vi "Quick Stack Get and Write Image.vi"(0 "Notifier Name":string, 7 "Write File Ref":refnum<file>, 11 "Num of Frames":u16) -> ()   [LabVIEW 2016]
uses:
  Device Library/Cameras/Camera Controls/Generic Camera Actions.ctl
  Device Library/Cameras/Camera Controls/Camera IMAQ Key Info.ctl
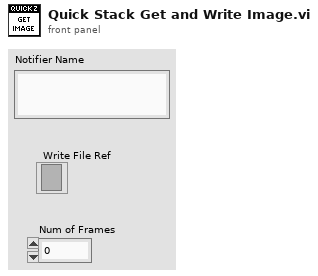
[diagram p1: front panel]
types:
  T1 = typedef "Camera IMAQ Key Info.ctl" = cluster{"Frame":u32, "Sensor Height":i32, "Sensor Width":i32, "ROI Height":i32, "ROI Width":i32, "ROI Enable?":bool, "Bit per Pixel":u8}
  T2 = typedef "Generic Camera Actions.ctl" = enum16{"Status", "Live Preview", "Capture", "Abort", "Set Exposure Time (s)", "Get Exposure Time (s)", "Record Settings", "Set ROI", "Get ROI", "Defect Correction On/Off", "Cooler On/Off", "Fan On/Off", "Quti"}
  T3 = typedef "IMAQ Image.ctl" = refnum<image>
  T4 = enum16{"big-endian, network order", "native, host order", "little-endian"}
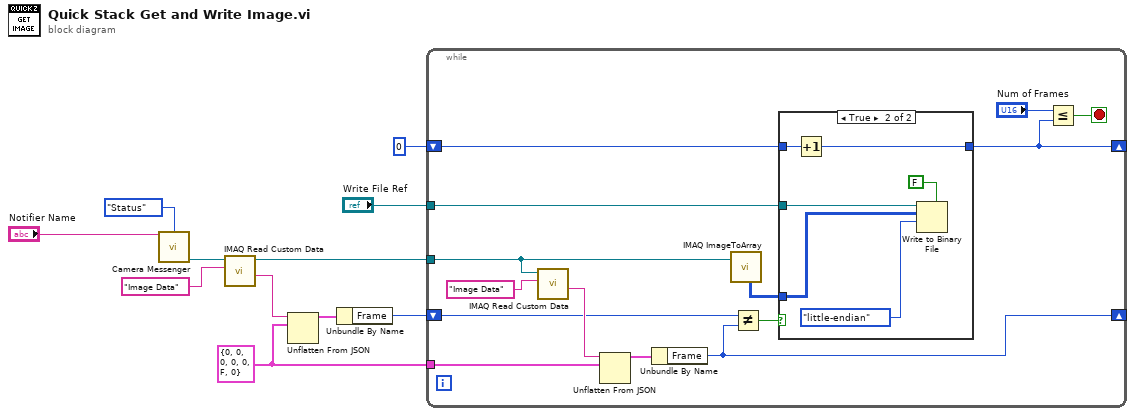
[diagram p0: block diagram]
diagram:
  w5 = T1 {"Frame"=0, "Sensor Height"=0, "Sensor Width"=0, "ROI Height"=0, "ROI Width"=0, "ROI Enable?"=FALSE, "Bit per Pixel"=0} ("Camera IMAQ Key Info")
  n1 = call "Camera Messenger.vi"("Notifier Name"="Notifier Name", "General Camera Actions"=Generic_Camera_Actions."Status") -> ("Image Ref"=w8:T3)  [unwired: 8 in, 5 out]
  n2 = call "IMAQ Read Custom Data"("Key"="Image Data", "Image"=w8) -> ("Custom Data Out"=w11:string, "Image (duplicate)"=w4:T3)  [unwired: 7 in, 1 out]
  n3 = Unflatten From JSON(JSON string=w11, type and defaults=w5) -> (value=w7:T1)  [unwired: 5 in, 1 out]
  n4 = Unbundle By Name(w7) -> ("Frame"=w6:u32)
  n5 = while {
    tunnel: w4 -> [w20]
    shift-right: [w15] -> _
    shift-left: w6 -> [w21]
    tunnel: w5 -> [w22]
    shift-right: [w14] -> _
    shift-left: u16 0 ("element") -> [w17]
    tunnel: "Write File Ref" -> [w16]
    stop <- w13 stop-if-true
    n6 = call "IMAQ Read Custom Data"("Key"="Image Data", "Image"=w20) -> ("Custom Data Out"=w24:string)  [unwired: 7 in, 2 out]
    n7 = Unflatten From JSON(JSON string=w24, type and defaults=w22) -> (value=w25:T1)  [unwired: 5 in, 1 out]
    n8 = Unbundle By Name(w25) -> ("Frame"=w15:u32)
    n9 = call "IMAQ ImageToArray"("Image"=w20) -> ("Image Pixels (U16)"=w18:u16[][])  [unwired: 3 in, 4 out]
    n10 = Not Equal?(x=w21, y=w15) -> (x != y?=w19:bool)
    n11 = case shown="True" w19 {
      tunnel: w18 -> [_ w28]
      tunnel: w17 -> [w26 w32]
      tunnel: [w26 w31] -> w14
      tunnel: w16 -> [_ w29]
      frame False {
      }
      frame True {
        n12 = Increment(x=w32) -> (x+1=w31:u16)
        n13 = Write to Binary File(file (use dialog)=w29, data=w28, 5:FALSE ("prepend array or string size? (T)"), 9:T4."little-endian" ("byte order (0:big-endian, network order)")) -> ()  [unwired: 2 in, 3 out]
      }
    }
    n14 = Less Or Equal?(x="Num of Frames", y=w14) -> (x <= y?=w13:bool)
  }
